vi "CtrlTreeAddDummyNodes.vi"(8 "error in (no error)":errorcluster, 9 "Dummy prefix":string="???? ", 10 "SavedSettings in":refnum<vi>, 11 "TreeControl in":refnum<vi>) -> (0 "error out":errorcluster, 3 "TreeControl out":refnum<vi>)   [LabVIEW 2019]
uses:
  b5c7daa3-e20d-4464-82b1-851610a55257.vi
  <vilib>/regexp/Match Regular Expression.xnode
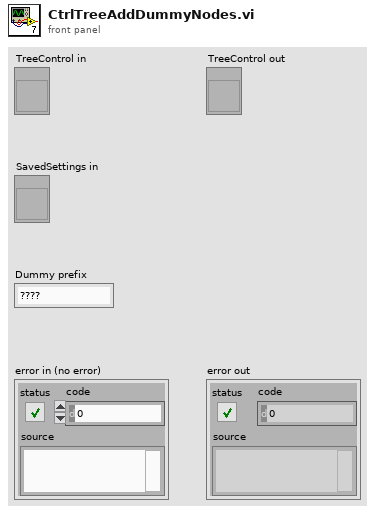
[diagram p1: front panel]
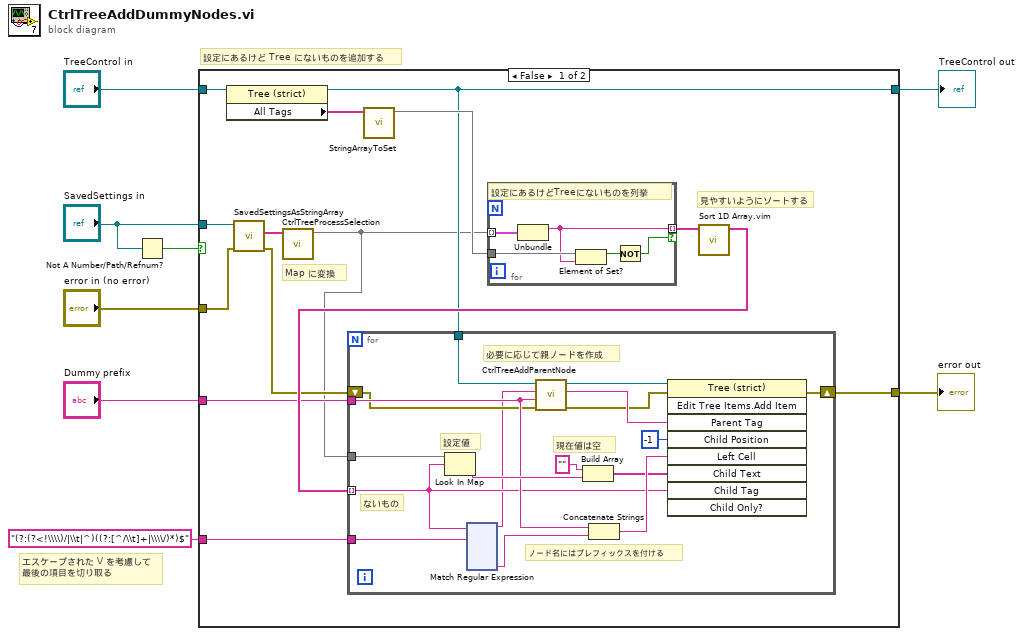
[diagram p0: block diagram]
diagram:
  # "エスケープされた \\/ を考慮して\n最後の項目を切り取る"
  # "設定にあるけど Tree にないものを追加する"
  n1 = Not A Number/Path/Refnum?(number/path/refnum="SavedSettings in") -> (NaN/Path/Refnum?=w2:bool)
  n2 = case shown="False" w2 {
    tunnel: "TreeControl in" -> [w20 w165]
    tunnel: [w11 w165] -> w4
    tunnel: "error in (no error)" -> [w14 w164]
    tunnel: [w12 w164] -> w6
    tunnel: "SavedSettings in" -> [w22 _]
    tunnel: "Dummy prefix" -> [w15 _]
    tunnel: "(?:(?<!\\\\)/|\\t|^)((?:[^/\\t]+|\\\\/)*)$" ("regular expression") -> [w9 _]
    frame False {
      # "見やすいようにソートする"
      # "Map に変換"
      n3 = property class="Tree (strict)"(reference=w20) -> (reference out=w11:refnum<vi>, "All Tags"=w17:string[])  [unwired: 1 in, 1 out]
      n4 = call "SavedSettingsAsStringArray.vi"("error in (no error)"=w14, "SavedSettings in"=w22) -> ("error out"=w13:errorcluster, "Selection"=w21:string[])  [unwired: 5 in, 3 out]
      n5 = call "CtrlTreeProcessSelection.vi"("Selection"=w21) -> ("Map"=w10:map{string, string})  [unwired: 10 in]
      n6 = call "StringArrayToSet.vi"("String Array"=w17) -> ("Set"=w16:set{string})  [unwired: 10 in]
      n7 = for {
        tunnel: w10 -> [w163] mode=indexing
        tunnel: [w159] -> w18 mode=indexing if=w160
        tunnel: w16 -> [w162]
        # "設定にあるけどTreeにないものを列挙"
        n8 = Unbundle(w163) -> (w159:string)  [unwired: 1 out]
        n9 = Element of Set?(10:w159, 11:w162) -> (3:w161:bool)
        n10 = Not(x=w161) -> (.not. x?=w160:bool)
      }
      n11 = call "Sort 1D Array.vim"("unsorted array"=w18) -> ("sorted array"=w19:string[])  [unwired: 10 in]
      n12 = for {
        tunnel: w19 -> [w26] mode=indexing
        tunnel: w10 -> [w35]
        tunnel: w15 -> [w31]
        shift-right: [w29] -> w12
        shift-left: w13 -> [w28]
        tunnel: w11 -> [w27]
        tunnel: w9 -> [w25]
        # "ノード名にはプレフィックスを付ける"
        # "必要に応じて親ノードを作成"
        # "現在値は空"
        # "設定値"
        # "ないもの"
        n13 = Look In Map(map=w35, key=w26) -> (value=w34:string)  [unwired: 1 in, 1 out]
        n14 = xnode "Match Regular Expression"("input string"=w26, "regular expression"=w25) -> ("before match"=w24:string, "submatch 1"=w23:string)  [unwired: 4 in, 4 out]
        n15 = call "CtrlTreeAddParentNode.vi"("error in (no error)"=w28, "Prefix"=w31, "Parent Tag"=w24, "TreeControl in"=w27) -> ("error out"=w30:errorcluster, "Tag out"=w33:string, "TreeControl out"=w32:refnum<vi>)  [unwired: 5 in]
        n16 = Build Array("", w34) -> (w37:string[])
        n17 = Concatenate Strings(w31, w23) -> (w39:string)
        n18 = invoke class="Tree (strict)" method="Edit Tree Items.Add Item"(reference=w32, error in=w30, "Parent Tag"=w33, "Child Position"=-1, "Left Cell"=w39, "Child Text"=w37, "Child Tag"=w26) -> (error out=w29:errorcluster)  [unwired: 2 in, 8 out]
      }
    }
    frame True {
    }
  }
  "error out" <- w6
  "TreeControl out" <- w4
